vi "5_ReleaseQueue.vi"(8 "error in (no error)":errorcluster caption="错误输入（无错误）", 11 "Queue In":refnum<queue>[](array[refnum])) -> (0 "error out":errorcluster caption="错误输出")   [LabVIEW 2017]
uses:
  Ctrls/QueueDataForm.ctl
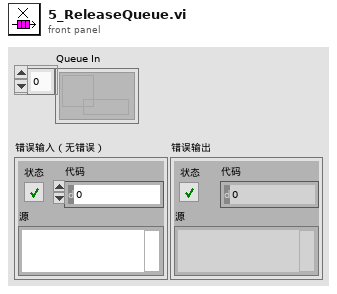
[diagram p1: front panel]
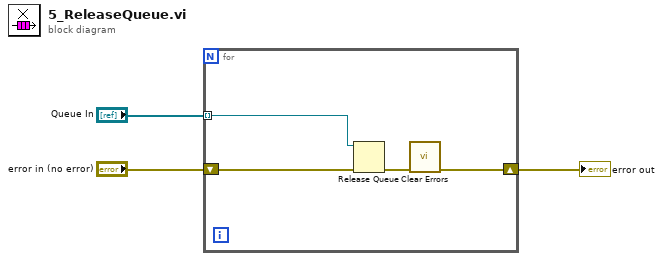
[diagram p0: block diagram]
diagram:
  n1 = for {
    tunnel: "Queue In" -> [w7] mode=indexing
    shift-right: [w4] -> w1
    shift-left: "error in (no error)" -> [w6]
    n2 = Release Queue(queue=w7, error in (no error)=w6) -> (error out=w5:errorcluster)  [unwired: 1 in, 2 out]
    n3 = call <vilib>:"Clear Errors.vi"("error in (no error)"=w5) -> ("error out"=w4:errorcluster)  [unwired: 5 in, 1 out]
  }
  "error out" <- w1
